vi "Get Interlock Status.vi"(8 "error in (no error)":errorcluster, 11 "VISA resource name":refnum<visa-resource-name>) -> (0 "error out":errorcluster, 2 "Interlock Asserted?":bool, 3 "VISA resource name out":refnum<visa-resource-name>)   [LabVIEW 2018, in "Keithley 2450.lvlib"]
doc: "This gives the status of the interlock.\n\nIf 1 is returned, the interlock signal is asserted and all voltage ranges are available.\nIf 0 is returned, the interlock is not asserted and the 200 V range is disabled. Lower voltage ranges are available."
uses:
  <instrlib>/Keithley 2450/Keithley 2450.lvlib
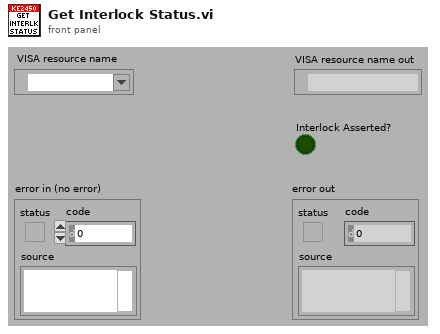
[diagram p1: front panel]
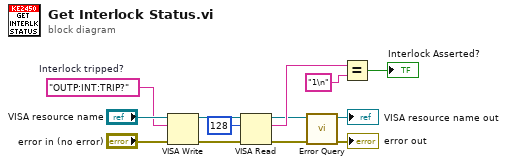
[diagram p0: block diagram]
diagram:
  w5 = "OUTP:INT:TRIP?"  # Interlock tripped?
  n1 = VISA Write(VISA resource name="VISA resource name", write buffer=w5, error in (no error)="error in (no error)") -> (VISA resource name out=w12:refnum<visa-resource-name>, error out=w13:errorcluster)  [unwired: 1 out]
  n2 = VISA Read(VISA resource name=w12, byte count=u32 128, error in (no error)=w13) -> (VISA resource name out=w2:refnum<visa-resource-name>, read buffer=w4:string, error out=w1:errorcluster)  [unwired: 1 out]
  n3 = call <instrlib>:"Error Query.vi"("error in (no error)"=w1, "VISA resource name"=w2) -> ("error out"=→"error out":errorcluster, "VISA resource name out"=→"VISA resource name out":refnum<visa-resource-name>)  [unwired: 8 out]
  n4 = Equal?(x=w4, y="1\n") -> (x = y?=→"Interlock Asserted?":bool)
